vi "CH_LM Register Event Callbacks.vi"(0 "CH_LM ActiveX Ref.":refnum<k7>, 11 "error in (no error)":errorcluster) -> (4 "dup CH_LM ActiveX Ref.":refnum<k7>, 6 "Event Callback refnum":refnum<k27>, 15 "error out":errorcluster)   [LabVIEW 2017, in "CH_LM.lvlib"]
doc: "This VI is used to register the LabMax ActiveX event callback VIs.\n\nFollowing LabMax ActiveX Events are supported:\n- MeterAdded\n- MeterRemoved\n- USBStreamingPacket\n- AsynchronousNotification"
uses:
  CH_LM.lvlib
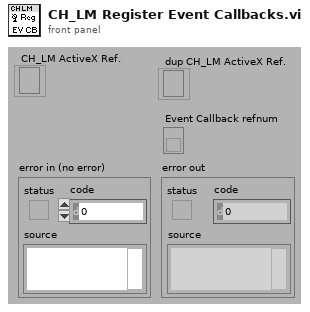
[diagram p1: front panel]
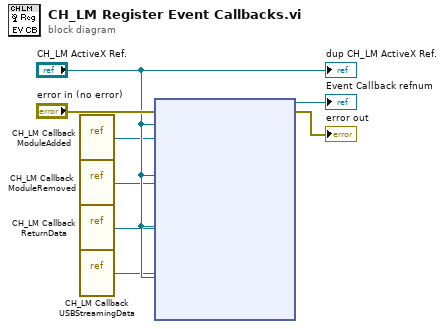
[diagram p0: block diagram]
diagram:
  n1 = vi-ref "CH_LM Callback ModuleAdded.vi"() -> ("vi reference"=w4:refnum<vi>)
  n2 = vi-ref "CH_LM Callback ModuleRemoved.vi"() -> ("vi reference"=w3:refnum<vi>)
  n3 = vi-ref "CH_LM Callback ReturnData.vi"() -> ("vi reference"=w2:refnum<vi>)
  n4 = vi-ref "CH_LM Callback USBStreamingData.vi"() -> ("vi reference"=w1:refnum<vi>)
  n5 = node ("Register Event Callback")("error in (no error)", "CH_LM ActiveX Ref.", w4, "CH_LM ActiveX Ref.", w3, "CH_LM ActiveX Ref.", w2, "CH_LM ActiveX Ref.", w1) -> (→"Event Callback refnum":refnum<k27>, →"error out":errorcluster)  [unwired: 5 in]
  "dup CH_LM ActiveX Ref." <- "CH_LM ActiveX Ref."
